vi "Cluster To Variant Attributes.vi"(0 "Variant of Cluster":variant, 1 "Base Indent":i32, 3 "Prefix":string, 5 "error in (no error)":errorcluster, 7 "Running Variant In":variant, 8 "If Empty":string="Cluster", 9 "Running Fields In":string[](array[string]), 11 "Running DataTypes In":T1[](array[typedef]), 13 "Running Indents In":i32[](array[numeric])) -> (14 "Variant Attributes Out":variant, 16 "Fields":string[](array[string]), 17 "DataTypes":T1[](array[typedef]), 18 "Indents":i32[](array[numeric]), 19 "error out":errorcluster)   [LabVIEW 2017, in "TreeLUT.lvclass"]
uses:
  TreeLUT.lvclass
  <vilib>/Utility/Data Type/Type Definitions/Data Type.ctl
  <vilib>/Utility/Data Type/NI_Data Type.lvlib
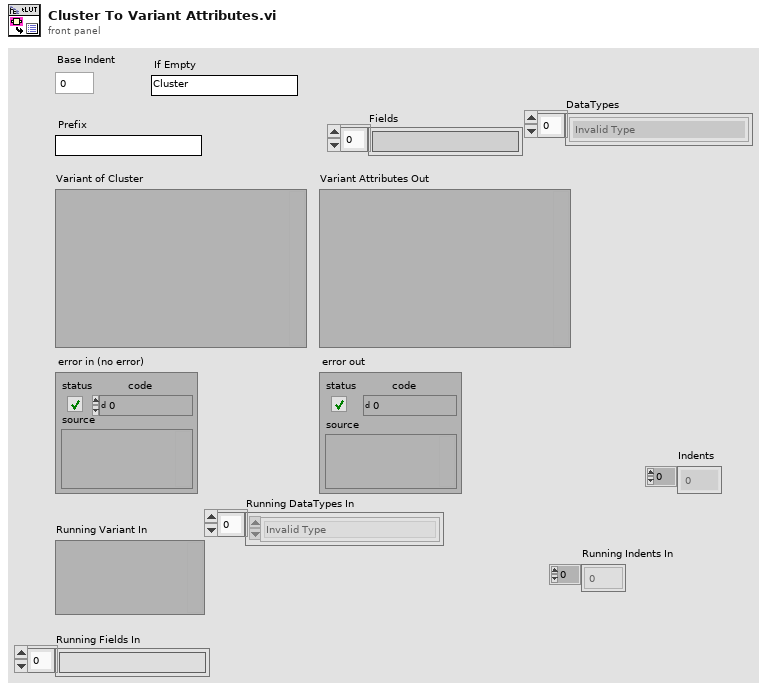
[diagram p1: front panel]
types:
  T1 = typedef "NI_Data Type.lvlib/Data Type.ctl" = enum8{"Invalid Type", "Void", "I8", "I16", "I32", "I64", "U8", "U16", "U32", "U64", "Single Float", "Double Float", "Extended Float", "Single Complex", "Double Complex", "Extended Complex", "Enum U8", "Enum U16", "Enum U32", "Enum U64", "Single Float With Unit", "Double Float With Unit", "Extended Float With Unit", "Single Complex with Unit", "Double Complex with Unit", "Extended Complex with Unit", "Boolean", "String", "Path", "Picture", "Tag", "Array", "Cluster", "Variant", "LV Variant", "Waveform", "Timestamp", "Digital Waveform", "Digital Data", "ExpressData", "Refnum", "External Data", "VI", "Poly VI", "LabVIEW Class Instance", "Fixed Point"}
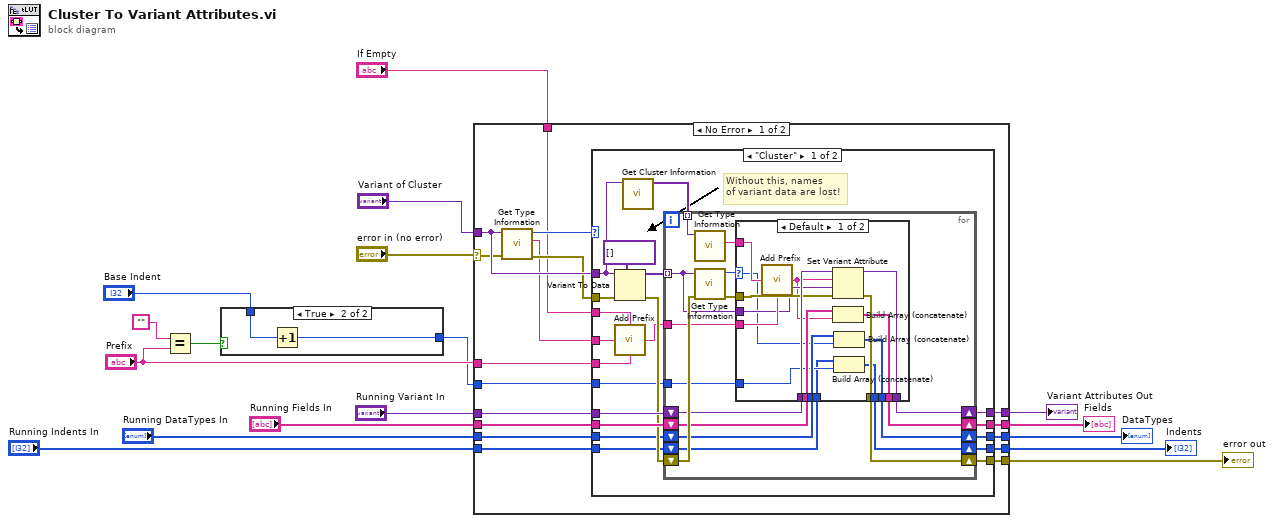
[diagram p0: block diagram]
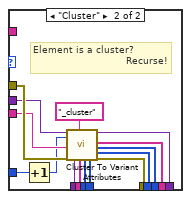
[diagram p3: hidden frame]
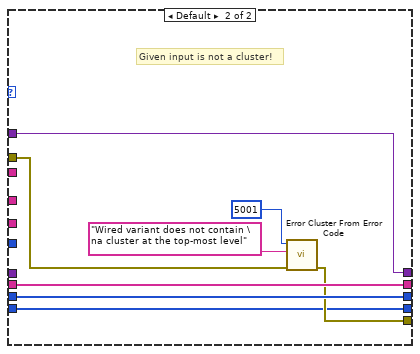
[diagram p4: hidden frame]
diagram:
  n1 = Equal?(x="", y="Prefix") -> (x = y?=w3:bool)
  n2 = case shown="True" w3 {
    tunnel: [w18 w19] -> w1
    tunnel: "Base Indent" -> [w18 w20]
    frame False {
    }
    frame True {
      n3 = Increment(x=w20) -> (x+1=w19:i32)
    }
  }
  n4 = case shown="No Error" "error in (no error)" {
    selector: "error in (no error)" -> [w34 w118]
    tunnel: [w32 w118] -> w16
    tunnel: "Variant of Cluster" -> [w36 w117]
    tunnel: "Running Variant In" -> [w35 _]
    tunnel: [w31 w117] -> w14
    tunnel: [w30 w116] -> w12
    tunnel: "Running Fields In" -> [w29 w116]
    tunnel: "Running DataTypes In" -> [w28 w115]
    tunnel: [w27 w115] -> w9
    tunnel: "Prefix" -> [w25 _]
    tunnel: "Running Indents In" -> [w24 w114]
    tunnel: [w23 w114] -> w7
    tunnel: w1 -> [w22 _]
    tunnel: "If Empty" -> [w21 _]
    frame No Error {
      n5 = call <vilib>:"Get Type Information.vi"("error in (no error)"=w34, "Variant"=w36) -> ("error out"=w33:errorcluster, "Name"=w26:string, "Type"=w37:T1)  [unwired: 5 in, 2 out]
      n6 = case shown="\"Cluster\"" w37 {
        tunnel: w36 -> [w48 w113]
        tunnel: w35 -> [w57 _]
        tunnel: w33 -> [w50 w109]
        tunnel: [w56 w110] -> w32
        tunnel: [w55 w113] -> w31
        tunnel: w29 -> [w52 w112]
        tunnel: [w51 w112] -> w30
        tunnel: w28 -> [w46 w111]
        tunnel: [w45 w111] -> w27
        tunnel: w26 -> [w44 _]
        tunnel: w25 -> [w43 _]
        tunnel: w24 -> [w41 w106]
        tunnel: [w40 w106] -> w23
        tunnel: w22 -> [w39 _]
        tunnel: w21 -> [w38 _]
        frame "Cluster" {
          # "Without this, names \nof variant data are lost!"
          n7 = Variant To Data(error in=w50, type=variant[] [], Variant=w48) -> (data=w53:variant[], error out=w49:errorcluster)
          n8 = call "Add Prefix.vi"("If Empty"=w38, "Name in"=w44, "Prefix"=w43) -> ("Name out"=w42:string)  [unwired: 12 in]
          n9 = call <vilib>:"Get Cluster Information.vi"("Variant"=w48) -> ("Cluster Elements"=w47:variant[])  [unwired: 9 in, 1 out]
          n10 = for {
            shift-right: [w69] -> w55
            shift-left: w57 -> [w70]
            tunnel: w42 -> [w72]
            tunnel: w53 -> [w65] mode=indexing
            shift-right: [w66] -> w51
            shift-left: w52 -> [w67]
            shift-right: [w68] -> w56
            shift-left: w49 -> [w74]
            tunnel: w47 -> [w64] mode=indexing
            shift-right: [w62] -> w45
            shift-left: w46 -> [w61]
            shift-right: [w59] -> w40
            shift-left: w41 -> [w60]
            tunnel: w39 -> [w58]
            n11 = call <vilib>:"Get Type Information.vi"("Variant"=w64) -> ("Name"=w63:string)  [unwired: 6 in, 4 out]
            n12 = call <vilib>:"Get Type Information.vi"("error in (no error)"=w74, "Variant"=w65) -> ("error out"=w71:errorcluster, "Type"=w73:T1)  [unwired: 5 in, 3 out]
            n13 = case shown="Default" w73 {
              selector: w73 -> [w78 _]
              tunnel: w72 -> [w85 w104]
              tunnel: w71 -> [w88 w105]
              tunnel: w70 -> [w90 w100]
              tunnel: [w89 w103] -> w69
              tunnel: w63 -> [w86 _]
              tunnel: [w87 w102] -> w68
              tunnel: w65 -> [w84 w101]
              tunnel: w67 -> [w83 w99]
              tunnel: [w82 w92] -> w66
              tunnel: [w80 w96] -> w62
              tunnel: w61 -> [w79 w98]
              tunnel: w60 -> [w76 w97]
              tunnel: [w75 w95] -> w59
              tunnel: w58 -> [w77 w94]
              frame Default {
                n14 = call "Add Prefix.vi"("Name in"=w86, "Prefix"=w85) -> ("Name out"=w81:string)  [unwired: 13 in]
                n15 = Set Variant Attribute(Variant=w90, name=w81, value=w84, error in=w88) -> (Variant out=w89:variant, error out=w87:errorcluster)  [unwired: 1 out]
                n16 = Build Array (concatenate)(w83, w81) -> (w82:string[])
                n17 = Build Array (concatenate)(w79, w78) -> (w80:T1[])
                n18 = Build Array (concatenate)(w76, w77) -> (w75:i32[])
              }
              frame "Cluster" {
                # "Element is a cluster?\n                               Recurse!"
                n19 = Increment(x=w94) -> (x+1=w93:i32)
                n20 = call "Cluster To Variant Attributes.vi"("Variant of Cluster"=w101, "Base Indent"=w93, "Prefix"=w104, "error in (no error)"=w105, "Running Variant In"=w100, "If Empty"="_cluster" ("Default IfEmpty"), "Running Fields In"=w99, "Running DataTypes In"=w98, "Running Indents In"=w97) -> ("Variant Attributes Out"=w103:variant, "Fields"=w92:string[], "DataTypes"=w96:T1[], "Indents"=w95:i32[], "error out"=w102:errorcluster)  [unwired: 6 in]
              }
            }
          }
        }
        frame Default {
          # "Given input is not a cluster!"
          n21 = call <vilib>:"Error Cluster From Error Code.vi"("error in (no error)"=w109, "error message (\"\")"="Wired variant does not contain \na cluster at the top-most level", "error code (0)"=5001) -> ("error out"=w110:errorcluster)  [unwired: 6 in]
        }
      }
    }
    frame Error {
    }
  }
  "Variant Attributes Out" <- w14
  "error out" <- w16
  "Fields" <- w12
  "DataTypes" <- w9
  "Indents" <- w7
